vi "Insert Word Into Little-Endian Bytes I16.vi"(6 "word":i16 format="%04x", 10 "index":i32, 11 "bytes":u8[](array[numeric]) format="%02x") -> (2 "index out":i32, 3 "bytes out":u8[](array[numeric]) format="%02x")   [LabVIEW 2020, in "NI_Bit Manipulation.lvlib"]
uses:
  <vilib>/Bit Manipulation/NI_Bit Manipulation.lvlib
  2b0808bd-7967-4d25-b8bc-26b4d176a5c8.vi
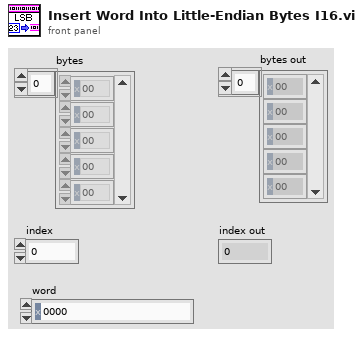
[diagram p1: front panel]
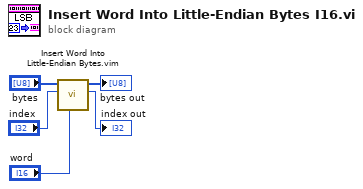
[diagram p0: block diagram]
diagram:
  n1 = call "Insert Word Into Little-Endian Bytes.vim"("word"="word", "index in"="index", "bytes in"="bytes") -> ("index out"=→"index out":i32, "bytes out"=→"bytes out":u8[])  [unwired: 7 in]
